vi "Hardware Message Loop.vi"(8 "error in":errorcluster, 10 "Data Notifier":refnum<notifier>, 11 "Message Queues":T8) -> (0 "error out":errorcluster)   [LabVIEW 2015, in "Hardware.lvlib"]
doc: "Message loop for handling messages pertaining to the acquisition of data from the hardware."
uses:
  Hardware.lvlib
  Support/Message Queue/All Message Queues.ctl
  Support/Message Queue/Message Cluster.ctl
  Scope data.ctl
  Settings/PFC Control settings.ctl
  PI Compensator.ctl
  Settings/Settings.ctl
  Settings/VSI Control settings.ctl
  Settings/PID Compensator.ctl
  Settings/Scope settings.ctl
  HW Rx State.ctl
  Acquisition State.ctl
  Support/Message Queue/Enqueue Message (Single).vi
  <vilib>/Utility/error.llb/Error Cluster From Error Code.vi
  <vilib>/ErrorRing/Error Ring.xnode
  Support/Message Queue/Message Queue.lvlib
  Settings/Settings.lvlib
panel:
  out "length 3":i32
  out "concatenated string 3":string
  out "VSI settings":T1={"FSM status"=enum."Stopped", "Ctrl bypass"=FALSE, "PID Control"={"Ref_val"=200.0, "Kp"=0.0, "Ti"=0.0, "Td"=0.0, "Out_min"=0.0, "Out_max"=0.0}, "3rd Harmonic"=FALSE, "Output enable"=FALSE, "Phase DBG"=2147} {"Phase DBG" format="%04x"}
  in  "start_rx":bool=TRUE
  out "return count":u32
  out "read buffer":string
  out "RX state":T3=enum."RX Header"
  out "Settings":T4={"HW Refnum"="USB0::0x0D7D::0x0100::2A49876D9CC1AA4::RAW", "PFC settings"={"FSM status"=enum."Stopped", "Voltage control ena"=FALSE, "Vea"=-1.0, "Voltage Ctrl bypass"=FALSE, "PI Voltage control"={"Ref_val"=0.0, "Kp"=0.0, "Ti"=0.0, "Out_min"=0.0, "Out_max"=0.0}, "Current Ctrl bypass"=FALSE, "PI Current control"={"Ref_val"=0.0, "Kp"=0.0, "Ti"=0.0, "Out_min"=0.0, "Out_max"=0.0}, "3rd Harmonic"=FALSE, "Output enable"=FALSE}, "VSI settings"={"FSM status"=enum."Stopped", "Ctrl bypass"=FALSE, "PID Control"={"Ref_val"=0.0, "Kp"=0.0, "Ti"=0.0, "Td"=0.0, "Out_min"=0.0, "Out_max"=0.0}, "3rd Harmonic"=FALSE, "Output enable"=FALSE, "Phase DBG"=0}, "Scope settings"={"run_stop"=FALSE, "single mode"=FALSE, "Trigger mode"=enum."Rising Edge", "Trigger source"=0, "trigger level"=0.0, "acq width"=100.0}} {"Scope settings"."Trigger source" items=["VLa", "VLb", "VLc"]; "Scope settings"."acq width" min=-12.0 max=12.0 step=1.0; "Scope settings"."trigger level" min=-12.0 max=12.0 step=1.0}
  out "PFC settings":T5={"FSM status"=enum."Stopped", "Voltage control ena"=FALSE, "Vea"=-1.0, "Voltage Ctrl bypass"=FALSE, "PI Voltage control"={"Ref_val"=0.0, "Kp"=0.0, "Ti"=0.0, "Out_min"=0.0, "Out_max"=0.0}, "Current Ctrl bypass"=FALSE, "PI Current control"={"Ref_val"=0.0, "Kp"=0.0, "Ti"=0.0, "Out_min"=0.0, "Out_max"=0.0}, "3rd Harmonic"=FALSE, "Output enable"=FALSE}
  out "concatenated string":string
  out "length":i32
  # "\"CTR:sendCfgVSI\""
  # "\"CTR:sendCfgPFC\""
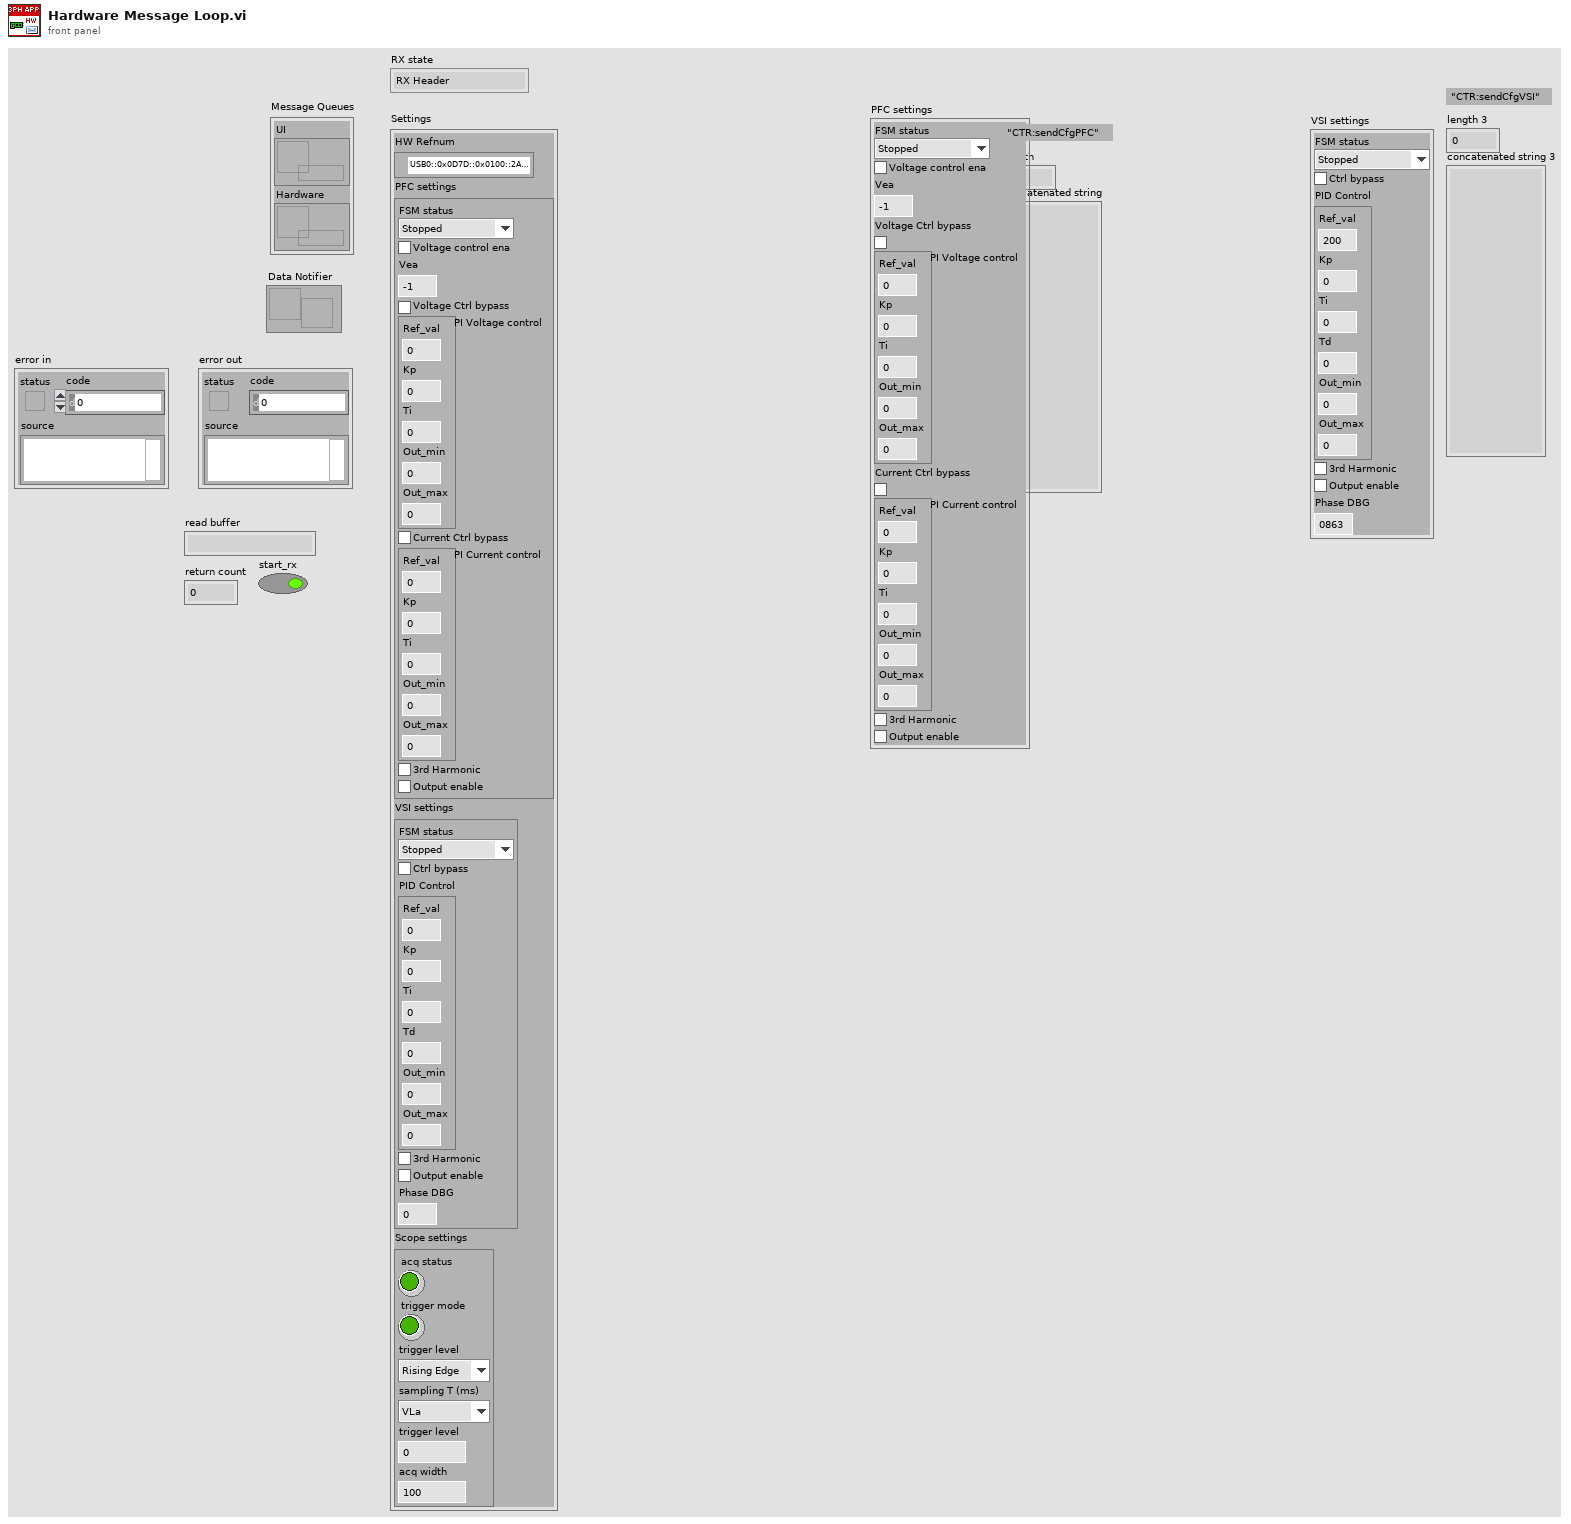
[diagram p1: front panel]
types:
  T1 = typedef "Settings.lvlib/VSI Control settings.ctl" = cluster{"FSM status":enum8{"Stopped", "Running"}, "Ctrl bypass":bool, "PID Control":T2, "3rd Harmonic":bool, "Output enable":bool, "Phase DBG":u32}
  T2 = typedef "Settings.lvlib/PID Compensator.ctl" = cluster{"Ref_val":sgl, "Kp":sgl, "Ti":sgl, "Td":sgl, "Out_min":sgl, "Out_max":sgl}
  T3 = typedef "Hardware.lvlib/HW Rx State.ctl" = enum16{"Idle", "RX Header", "RX Scope cargo", "RX Control cfg cargo", "Exit"}
  T4 = typedef "Settings.lvlib/Settings.ctl" = cluster{"HW Refnum":refnum<visa-resource-name>, "PFC settings":T5, "VSI settings":T1, "Scope settings":T7}
  T5 = typedef "Settings.lvlib/PFC Control settings.ctl" = cluster{"FSM status":enum8{"Stopped", "Running"}, "Voltage control ena":bool, "Vea":sgl, "Voltage Ctrl bypass":bool, "PI Voltage control":T6, "Current Ctrl bypass":bool, "PI Current control":T6, "3rd Harmonic":bool, "Output enable":bool}
  T6 = typedef "Settings.lvlib/PI Compensator.ctl" = cluster{"Ref_val":sgl, "Kp":sgl, "Ti":sgl, "Out_min":sgl, "Out_max":sgl}
  T7 = typedef "Settings.lvlib/Scope settings.ctl" = cluster{"run_stop":bool, "single mode":bool, "Trigger mode":enum16{"Auto", "Rising Edge", "Falling Edge", "Both Edges"}, "Trigger source":u16, "trigger level":dbl, "acq width":dbl}
  T8 = typedef "Message Queue.lvlib/All Message Queues.ctl" = cluster{"UI":refnum<queue>, "Hardware":refnum<queue>}
  T9 = typedef "Hardware.lvlib/Acquisition State.ctl" = enum16{"Idle", "Acquiring"}
  T10 = typedef "Hardware.lvlib/Packet type.ctl" = enum16{"Null", "Scope data", "Control cfg echo"}
  T11 = typedef "Hardware.lvlib/Scope data.ctl" = cluster{"IS_DC_IN":dbl[], "VS_DC_IN":dbl[], "IS_DC_OUT":dbl[], "VS_DC_OUT":dbl[], "VS_La":dbl[], "VS_Lb":dbl[], "VS_Lc":dbl[], "IS_La":dbl[], "IS_Lb":dbl[], "IS_Lc":dbl[], "Vea":i16[], "da":i16[], "db":i16[], "dc":i16[], "alfa_ref":dbl[], "i_alfa":dbl[]}
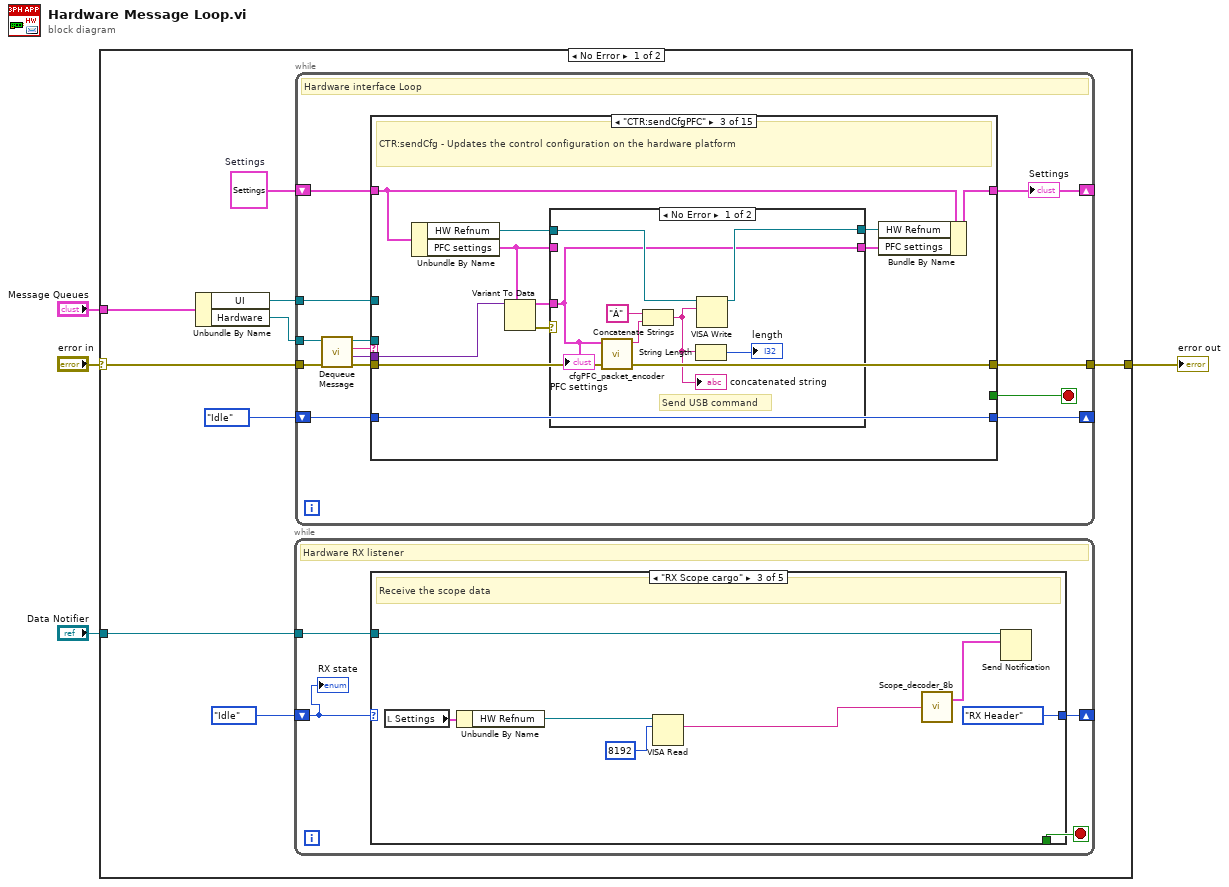
[diagram p0: block diagram]
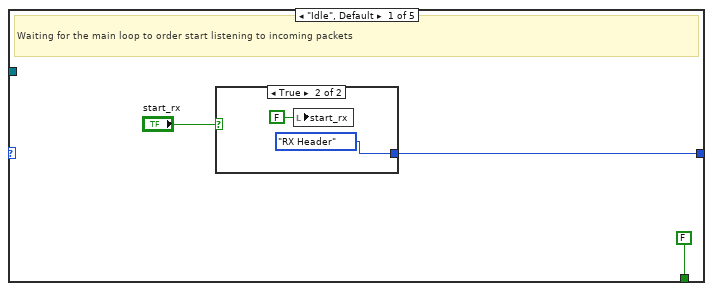
[diagram p2: hidden frame]
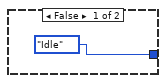
[diagram p3: hidden frame]
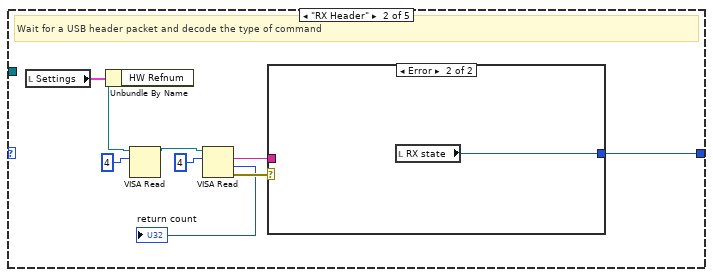
[diagram p4: hidden frame]
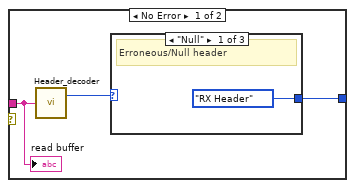
[diagram p5: hidden frame]
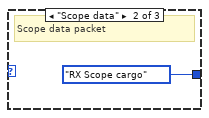
[diagram p6: hidden frame]
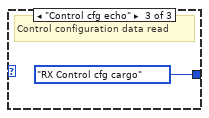
[diagram p7: hidden frame]
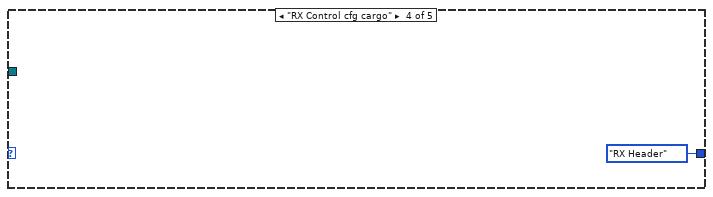
[diagram p8: hidden frame]
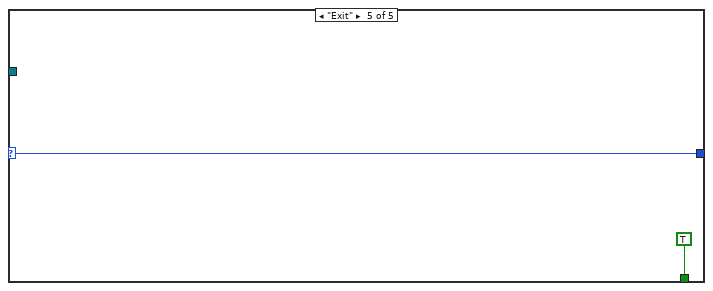
[diagram p9: hidden frame]
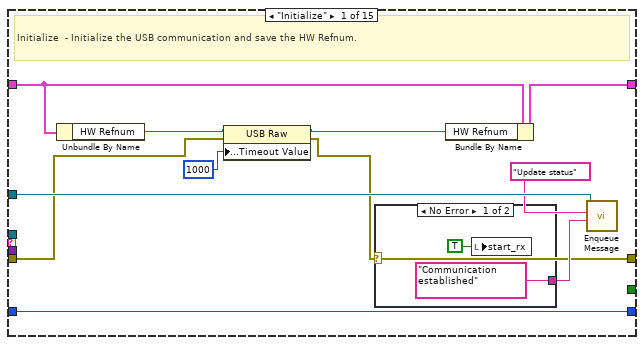
[diagram p10: hidden frame]
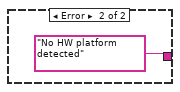
[diagram p11: hidden frame]
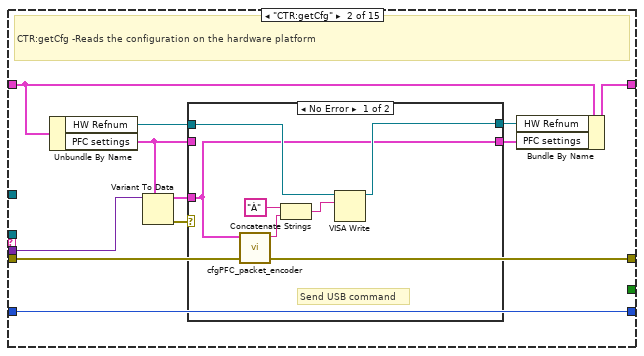
[diagram p12: hidden frame]
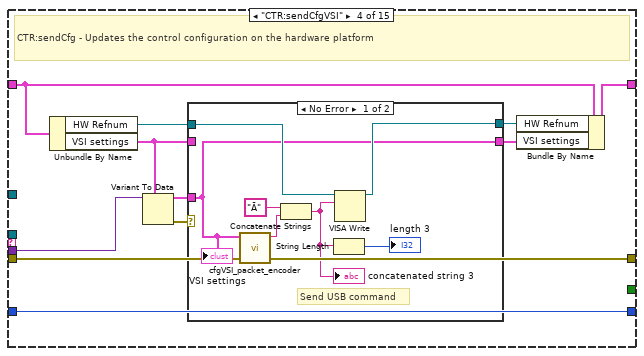
[diagram p15: hidden frame]
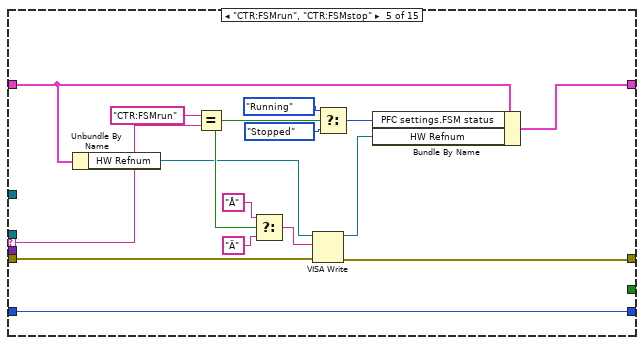
[diagram p17: hidden frame]
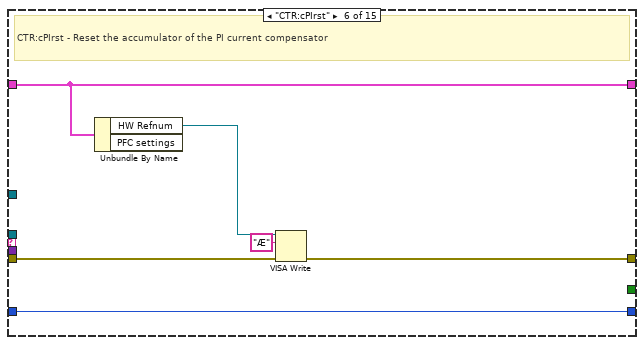
[diagram p18: hidden frame]
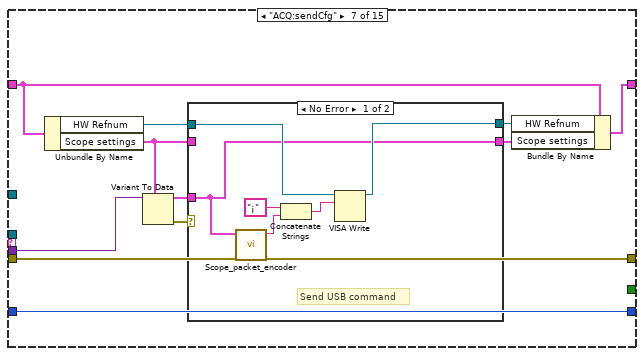
[diagram p19: hidden frame]
diagram:
  n1 = case shown="No Error" "error in" {
    selector: "error in" -> [w10 w257]
    tunnel: "Message Queues" -> [w13 _]
    tunnel: [w11 w257] -> w3
    tunnel: "Data Notifier" -> [w7 _]
    frame No Error {
      w5 = T4 {"HW Refnum"="USB0::0x0D7D::0x0100::2A49876D9CC1AA4::RAW", "PFC settings"={"FSM status"=enum."Stopped", "Voltage control ena"=FALSE, "Vea"=0.0, "Voltage Ctrl bypass"=FALSE, "PI Voltage control"={"Ref_val"=0.0, "Kp"=0.0, "Ti"=0.0, "Out_min"=0.0, "Out_max"=0.0}, "Current Ctrl bypass"=FALSE, "PI Current control"={"Ref_val"=0.0, "Kp"=0.0, "Ti"=0.0, "Out_min"=0.0, "Out_max"=0.0}, "3rd Harmonic"=FALSE, "Output enable"=FALSE}, "VSI settings"={"FSM status"=enum."Stopped", "Ctrl bypass"=FALSE, "PID Control"={"Ref_val"=0.0, "Kp"=0.0, "Ti"=0.0, "Td"=0.0, "Out_min"=0.0, "Out_max"=0.0}, "3rd Harmonic"=FALSE, "Output enable"=FALSE, "Phase DBG"=0}, "Scope settings"={"run_stop"=FALSE, "single mode"=FALSE, "Trigger mode"=enum."Auto", "Trigger source"=0, "trigger level"=0.0, "acq width"=0.0}}  # Settings
      n2 = Unbundle By Name(w13) -> ("UI"=w9:refnum<queue>, "Hardware"=w12:refnum<queue>)
      n3 = while {
        tunnel: w7 -> [w17]
        shift-right: [w16] -> _
        shift-left: HW_Rx_State."Idle" ("State") -> [w14]
        stop <- w15 stop-if-true
        # "Hardware RX listener"
        n4 = case shown="\"RX Scope cargo\"" w14 {
          selector: w14 -> [_ _ _ _ w48]
          tunnel: [w18 w31 HW_Rx_State."RX Header" ("State") HW_Rx_State."RX Header" ("State") w48] -> w16
          tunnel: w17 -> [_ _ w45 _ _]
          tunnel: [FALSE _ _ _ TRUE] -> w15
          frame "Idle", Default {
            # "Waiting for the main loop to order start listening to incoming packets"
            n5 = case shown="True" "start_rx" {
              tunnel: [HW_Rx_State."Idle" ("State") HW_Rx_State."RX Header" ("State")] -> w18
              frame False {
              }
              frame True {
                n6 = local write "start_rx"(FALSE ("start_rx")) -> ()
              }
            }
          }
          frame "RX Header" {
            # "Wait for a USB header packet and decode the type of command"
            n7 = local read "Settings"() -> (w32:T4)
            n8 = Unbundle By Name(w32) -> ("HW Refnum"=w24:refnum<visa-resource-name>)
            n9 = VISA Read(VISA resource name=w24, byte count=u32 4) -> (VISA resource name out=w25:refnum<visa-resource-name>)  [unwired: 1 in, 3 out]
            n10 = VISA Read(VISA resource name=w25, byte count=u32 4) -> (read buffer=w29:string, return count=→"return count":u32, error out=w28:errorcluster)  [unwired: 1 in, 1 out]
            n11 = case shown="Error" w28 {
              tunnel: [w35 w39] -> w31
              tunnel: w29 -> [w34 _]
              frame No Error {
                n12 = call "Header_decoder.vi"("header"=w34) -> ("Type"=w33:T10)  [unwired: 1 out]
                n13 = case shown="\"Null\"" w33 {
                  tunnel: [HW_Rx_State."RX Header" ("State") HW_Rx_State."RX Scope cargo" ("State") HW_Rx_State."RX Control cfg cargo" ("State")] -> w35
                  frame "Null" {
                    # "Erroneous/Null header"
                  }
                  frame "Scope data" {
                    # "Scope data packet"
                  }
                  frame "Control cfg echo" {
                    # "Control configuration data read"
                  }
                }
                "read buffer" <- w34
              }
              frame Error {
                n14 = local read "RX state"() -> (w39:T3)
              }
            }
          }
          frame "RX Scope cargo" {
            # "Receive the scope data"
            n15 = local read "Settings"() -> (w46:T4)
            n16 = Unbundle By Name(w46) -> ("HW Refnum"=w41:refnum<visa-resource-name>)
            n17 = VISA Read(VISA resource name=w41, byte count=u32 8192) -> (read buffer=w40:string)  [unwired: 1 in, 3 out]
            n18 = call "Scope_decoder_8b.vi"("raw_data"=w40) -> ("scope_data"=w43:T11)  [unwired: 1 in]
            n19 = Send Notification(notification=w43, notifier=w45) -> ()  [unwired: 1 in, 2 out]
          }
          frame "RX Control cfg cargo" {
          }
          frame "Exit" {
          }
        }
        "RX state" <- w14
      }
      n20 = while {
        tunnel: w12 -> [w56]
        shift-right: [w50] -> _
        shift-left: w5 -> [w62]
        tunnel: w9 -> [w52]
        shift-right: [w54] -> _
        shift-left: Acquisition_State."Idle" ("State") -> [w55]
        tunnel: w10 -> [w60]
        tunnel: [w51] -> w11
        stop <- w61 stop-if-true
        # "Hardware interface Loop"
        n21 = call "Dequeue Message.vi"("error in (no error)"=w60, "Message Queue"=w56) -> ("error out"=w59:errorcluster, "Message Data"=w57:variant, "Message"=w58:string, "dup Message Queue"=w53:refnum<queue>)  [unwired: 6 in]
        n22 = case "Message Cases" shown="\"CTR:sendCfgPFC\"" w58 {
          selector: w58 -> [_ _ _ _ w149 _ _ _ _ _ _ _ _ _ w246]
          tunnel: w53 -> [_ _ _ _ _ _ _ _ _ _ _ w214 _ w244 _]
          tunnel: w59 -> [w65 w87 w106 w126 w144 w152 w158 w184 w190 w200 w208 w213 w227 w237 _]
          tunnel: [w63 w87 w106 w126 w143 w153 w158 w180 w192 w196 w204 w215 w233 w242 w247] -> w51
          tunnel: w62 -> [w71 w81 w100 w120 w137 w156 w161 w182 w191 w198 w206 w211 w229 w238 w249]
          tunnel: [w72 w80 w99 w119 w150 w156 w162 w181 w189 w197 w205 w212 w228 w238 w249] -> w50
          tunnel: [_ _ _ _ _ _ _ _ _ _ _ _ _ TRUE _] -> w61
          tunnel: w57 -> [_ w85 w104 w124 _ _ w160 _ _ _ _ _ w232 _ _]
          tunnel: w52 -> [w70 _ _ _ _ _ _ _ _ _ _ _ _ _ _]
          tunnel: w55 -> [w73 w86 w105 w125 w151 w157 w159 _ _ _ _ w209 w226 w243 w248]
          tunnel: [w73 w86 w105 w125 w151 w157 w159 Acquisition_State."Idle" ("State") Acquisition_State."Acquiring" ("Acquisition State") Acquisition_State."Idle" ("State") Acquisition_State."Idle" ("State") w210 w226 w243 w248] -> w54
          frame "Initialize" {
            # "Initialize  - Initialize the USB communication and save the HW Refnum."
            n23 = Unbundle By Name(w71) -> ("HW Refnum"=w66:refnum<visa-resource-name>)
            n24 = property on="Property Node" class="USB Raw"(reference=w66, error in=w65, "General Settings:Timeout Value"=u32 1000) -> (reference out=w64:refnum<visa-resource-name>, error out=w63:errorcluster)
            n25 = case shown="No Error" w63 {
              tunnel: ["Communication established" ("Message") "No HW platform detected" ("Message")] -> w68
              frame No Error {
                n26 = local write "start_rx"(TRUE ("start_rx")) -> ()
              }
              frame Error {
              }
            }
            n27 = Bundle By Name(cluster=w71, "HW Refnum"=w64) -> (w72:T4)
            n28 = call-poly "Enqueue Message.vi"("Message Data"=w68, "Message"="Update status", "Message Queue"=w70) -> ()  [unwired: 7 in, 2 out]
          }
          frame "CTR:getCfg" {
            # "CTR:getCfg -Reads the configuration on the hardware platform"
            n29 = Unbundle By Name(w81) -> ("HW Refnum"=w78:refnum<visa-resource-name>, "PFC settings"=w82:T5)
            n30 = Variant To Data(type=w82, Variant=w85) -> (data=w79:T5, error out=w84:errorcluster)  [unwired: 1 in]
            n31 = case shown="No Error" w84 {
              tunnel: [w91 w95] -> w83
              tunnel: w82 -> [_ w95]
              tunnel: w79 -> [w91 _]
              tunnel: w78 -> [w93 w94]
              tunnel: [w92 w94] -> w77
              frame No Error {
                # "Send USB command"
                n32 = call "cfgPFC_packet_encoder.vi"("Control settings"=w91) -> ("concatenated string"=w89:string)  [unwired: 10 in]
                n33 = Concatenate Strings("À" ("write buffer"), w89) -> (w88:string)
                n34 = VISA Write(VISA resource name=w93, write buffer=w88) -> (VISA resource name out=w92:refnum<visa-resource-name>)  [unwired: 1 in, 2 out]
              }
              frame Error {
              }
            }
            n35 = Bundle By Name(cluster=w81, "HW Refnum"=w77, "PFC settings"=w83) -> (w80:T4)
          }
          frame "CTR:sendCfgPFC" {
            # "CTR:sendCfg - Updates the control configuration on the hardware platform"
            n36 = Unbundle By Name(w100) -> ("HW Refnum"=w97:refnum<visa-resource-name>, "PFC settings"=w101:T5)
            n37 = Variant To Data(type=w101, Variant=w104) -> (data=w98:T5, error out=w103:errorcluster)  [unwired: 1 in]
            n38 = case shown="No Error" w103 {
              tunnel: [w110 w115] -> w102
              tunnel: w101 -> [_ w115]
              tunnel: w98 -> [w110 _]
              tunnel: w97 -> [w113 w114]
              tunnel: [w112 w114] -> w96
              frame No Error {
                # "Send USB command"
                n39 = call "cfgPFC_packet_encoder.vi"("Control settings"=w110) -> ("concatenated string"=w108:string)  [unwired: 10 in]
                n40 = Concatenate Strings("Á" ("write buffer"), w108) -> (w107:string)
                "concatenated string" <- w107
                n41 = String Length(string=w107) -> (length=→"length":i32)
                n42 = VISA Write(VISA resource name=w113, write buffer=w107) -> (VISA resource name out=w112:refnum<visa-resource-name>)  [unwired: 1 in, 2 out]
                "PFC settings" <- w110
              }
              frame Error {
              }
            }
            n43 = Bundle By Name(cluster=w100, "HW Refnum"=w96, "PFC settings"=w102) -> (w99:T4)
          }
          frame "CTR:sendCfgVSI" {
            # "CTR:sendCfg - Updates the control configuration on the hardware platform"
            n44 = Unbundle By Name(w120) -> ("HW Refnum"=w117:refnum<visa-resource-name>, "VSI settings"=w121:T1)
            n45 = Variant To Data(type=w121, Variant=w124) -> (data=w118:T1, error out=w123:errorcluster)  [unwired: 1 in]
            n46 = case shown="No Error" w123 {
              tunnel: [w130 w135] -> w122
              tunnel: w121 -> [_ w135]
              tunnel: w118 -> [w130 _]
              tunnel: w117 -> [w133 w134]
              tunnel: [w132 w134] -> w116
              frame No Error {
                # "Send USB command"
                n47 = call "cfgVSI_packet_encoder.vi"("Control settings"=w130) -> ("concatenated string"=w128:string)  [unwired: 10 in]
                n48 = Concatenate Strings("Ã" ("write buffer"), w128) -> (w127:string)
                "concatenated string 3" <- w127
                n49 = String Length(string=w127) -> (length=→"length 3":i32)
                n50 = VISA Write(VISA resource name=w133, write buffer=w127) -> (VISA resource name out=w132:refnum<visa-resource-name>)  [unwired: 1 in, 2 out]
                "VSI settings" <- w130
              }
              frame Error {
              }
            }
            n51 = Bundle By Name(cluster=w120, "HW Refnum"=w116, "VSI settings"=w122) -> (w119:T4)
          }
          frame "CTR:FSMrun", "CTR:FSMstop" {
            n52 = Unbundle By Name(w137) -> ("HW Refnum"=w136:refnum<visa-resource-name>)
            n53 = Equal?(x="CTR:FSMrun", y=w149) -> (x = y?=w139:bool)
            n54 = Select(t="Å" ("write buffer"), s=w139, f="Ä" ("write buffer")) -> (s? t:f=w142:string)
            n55 = VISA Write(VISA resource name=w136, write buffer=w142, error in (no error)=w144) -> (VISA resource name out=w138:refnum<visa-resource-name>, error out=w143:errorcluster)  [unwired: 1 out]
            n56 = Select(t=enum16{"Stopped", "Running"}."Running" ("Control settings.FSM status"), s=w139, f=enum16{"Stopped", "Running"}."Stopped" ("Control settings.FSM status")) -> (s? t:f=w146:enum16{"Stopped", "Running"})
            n57 = Bundle By Name(cluster=w137, "PFC settings.FSM status"=w146, "HW Refnum"=w138) -> (w150:T4)
          }
          frame "CTR:cPIrst" {
            # "CTR:cPIrst - Reset the accumulator of the PI current compensator"
            n58 = Unbundle By Name(w156) -> ("HW Refnum"=w155:refnum<visa-resource-name>)  [unwired: 1 out]
            n59 = VISA Write(VISA resource name=w155, write buffer="Æ", error in (no error)=w152) -> (error out=w153:errorcluster)  [unwired: 2 out]
          }
          frame "ACQ:sendCfg" {
            n60 = Unbundle By Name(w161) -> ("HW Refnum"=w164:refnum<visa-resource-name>, "Scope settings"=w166:T7)
            n61 = Variant To Data(type=w166, Variant=w160) -> (data=w165:T7, error out=w168:errorcluster)  [unwired: 1 in]
            n62 = case shown="No Error" w168 {
              tunnel: [w170 w176] -> w167
              tunnel: w166 -> [_ w176]
              tunnel: w165 -> [w170 _]
              tunnel: w164 -> [w174 w175]
              tunnel: [w173 w175] -> w163
              frame No Error {
                # "Send USB command"
                n63 = call "Scope_packet_encoder.vi"("Scope settings"=w170) -> ("concatenated string"=w169:string)  [unwired: 10 in]
                n64 = Concatenate Strings("¡" ("write buffer"), w169) -> (w171:string)
                n65 = VISA Write(VISA resource name=w174, write buffer=w171) -> (VISA resource name out=w173:refnum<visa-resource-name>)  [unwired: 1 in, 2 out]
              }
              frame Error {
              }
            }
            n66 = Bundle By Name(cluster=w161, "HW Refnum"=w163, "Scope settings"=w167) -> (w162:T4)
          }
          frame "ACQ:stop" {
            # "Stop - Stop the Acquisition."
            n67 = Unbundle By Name(w182) -> ("HW Refnum"=w178:refnum<visa-resource-name>)
            n68 = VISA Write(VISA resource name=w178, write buffer="¢", error in (no error)=w184) -> (VISA resource name out=w177:refnum<visa-resource-name>, error out=w180:errorcluster)  [unwired: 1 out]
            n69 = Bundle By Name(cluster=w182, "HW Refnum"=w177) -> (w181:T4)
          }
          frame "ACQ:run" {
            # "ACQ:run - Configure and start the acquisition."
            n70 = Unbundle By Name(w191) -> ("HW Refnum"=w186:refnum<visa-resource-name>)
            n71 = VISA Write(VISA resource name=w186, write buffer="£", error in (no error)=w190) -> (VISA resource name out=w185:refnum<visa-resource-name>, error out=w192:errorcluster)  [unwired: 1 out]
            n72 = Bundle By Name(cluster=w191, "HW Refnum"=w185) -> (w189:T4)
          }
          frame "ACQ:singleRST" {
            # "ACQ:singleRST - Set the scope to SINGLE mode."
            n73 = Unbundle By Name(w198) -> ("HW Refnum"=w194:refnum<visa-resource-name>)
            n74 = VISA Write(VISA resource name=w194, write buffer="¤", error in (no error)=w200) -> (VISA resource name out=w193:refnum<visa-resource-name>, error out=w196:errorcluster)  [unwired: 1 out]
            n75 = Bundle By Name(cluster=w198, "HW Refnum"=w193) -> (w197:T4)
          }
          frame "ACQ:singleSET" {
            # "ACQ:singleSET - Set the scope to SINGLE mode."
            n76 = Unbundle By Name(w206) -> ("HW Refnum"=w202:refnum<visa-resource-name>)
            n77 = VISA Write(VISA resource name=w202, write buffer="¥", error in (no error)=w208) -> (VISA resource name out=w201:refnum<visa-resource-name>, error out=w204:errorcluster)  [unwired: 1 out]
            n78 = Bundle By Name(cluster=w206, "HW Refnum"=w201) -> (w205:T4)
          }
          frame "Acquire" {
            # "Acquire - Acquire data from the hardware. Since this is a continuous acquisition, this message will always message itself to run again."
            n79 = case shown="\"Acquiring\"" w209 {
              selector: w209 -> [w216 w221]
              tunnel: [w217 w225] -> w215
              tunnel: w214 -> [_ w223]
              tunnel: w213 -> [w217 w220]
              tunnel: [w218 w219] -> w212
              tunnel: w211 -> [w218 w219]
              tunnel: [w216 w221] -> w210
              frame "Idle" {
                # "Ignore \"Acquire\" messages when the acquisition is idle."
              }
              frame "Acquiring" {
                # "Acquire data while in the \"Acquiring\" state."
                n80 = call-poly "Enqueue Message.vi"("error in (no error)"=w220, "Message"="Acquire", "Message Queue"=w223) -> ("error out"=w224:errorcluster)  [unwired: 7 in, 1 out]
                n81 = Merge Errors(w224) -> (w225:errorcluster)
              }
            }
          }
          frame "Update Settings" {
            # "New settings are available, update the current ones stored in the shift register with the settings sent as part of the message"
            n82 = Variant To Data(error in=w227, type=w229, Variant=w232) -> (data=w230:T4, error out=w231:errorcluster)
            n83 = Select(t=w229, s=w231, f=w230) -> (s? t:f=w228:T4)
            n84 = Merge Errors(w227) -> (w233:errorcluster)
          }
          frame "Exit" {
            # "Release the Acquisition queue reference"
            # "Stop the VI"
            # "Exit - Close the comunication with the HW platform and exit the VI."
            n85 = Unbundle By Name(w238) -> ("HW Refnum"=w239:refnum<visa-resource-name>)
            n86 = VISA Write(VISA resource name=w239, write buffer="\u0011", error in (no error)=w237) -> (VISA resource name out=w236:refnum<visa-resource-name>, error out=w235:errorcluster)  [unwired: 1 out]
            n87 = VISA Close(VISA resource name=w236, error in (no error)=w235) -> (error out=w234:errorcluster)
            n88 = local write "RX state"(HW_Rx_State."Exit" ("RX state")) -> ()
            n89 = Release Queue(queue=w244, error in (no error)=w234) -> (error out=w242:errorcluster)  [unwired: 1 in, 2 out]
          }
          frame Default {
            # "'Default' case only runs if there is a message that isn't defined in any of the other cases.  Output a programming error."
            n90 = xnode "Error Ring"("parameter 0"=w246) -> ("error out"=w247:errorcluster)
          }
        }
        "Settings" <- w50
      }
    }
    frame Error {
    }
  }
  "error out" <- w3
